vi "Type_3.vi"(7 "프런트패널 윈도우:동작":T1(ring)=enum."Default", 8 "에러 입력":errorcluster caption="에러 입력(에러 없음)", 11 "세부분류코드":string caption="확장자없는 파일 이름") -> (0 "error out":errorcluster)   [LabVIEW 2020]
uses:
  Support/Controls/Cmd_Mouse Popup.ctl
  Support/Controls/Clst_Query Info.ctl
  Support/Controls/Cmd_Read Query.ctl
  Support/Public/Polymorph/Array Dedup_1D Str.vi
  Support/Public/Polymorph/Cell Space_Table.vi
  <vilib>/addons/database/NI_Database_API.lvlib
panel:
  in  "탭 컨트롤":enum32{"검색", "등록", "CMC"}(tab)
  in  "일부추가":bool
  in  "최소범위검색":bool
  in  "최소 범위 검색":dbl
  in  "Condition_2":i32(listbox) caption="최소 측정 범위"
  out "인정범위":string[][](table)
  out "SQL Quary 컬럼명":string
  out "Calfunc":string[][](array[string])
  out "모델정보":string[][](array[string])
  in  "옵션검색":bool
  in  "옵션 검색 조건":string(combo)
  in  "모델검색":bool
  in  "모델 검색 조건":string
  in  "최대범위검색":bool
  in  "최대 범위 검색":dbl
  in  "전체추가":bool
  out "소분류코드":string
  out "측정기명":string
  in  "Condition_1":i32(listbox) caption="최대 측정 범위"
  in  "모델 및 옵션 List":i32(listbox)
  out "Load Proc":string[][](table) caption="등록된 교정 Procedure"
  in  "교정기능":string(combo)
  in  "구분 2":string(combo) caption="엑셀파일명"
  in  "참고 버튼":bool
  in  "교정값":string
  in  "명목값":string caption="명목값 (호칭)"
  in  "추가단위":string(combo)="mg" caption="단위"
  in  "구분":string(combo) caption="측정방식"
  out "Func_ext ?":bool
  out "배열":u32[](array[numeric])
  in  "단위":string(combo)
  in  "변경 버튼":bool
  in  "등록 버튼":bool
  in  "교정점 추가 버튼":bool
  in  "교정점":string
  in  "Proc":string[][](table) caption="등록할 교정 Procedure"
  in  "형식":string
  in  "옵션":string
  in  "최소눈금":string(combo)
  in  "교정기능 2":string(combo) caption="교정기능"
  in  "표시방식":string(combo)
  out "CMC":string[][](table)
  # "항목정보"
  # "검색옵션"
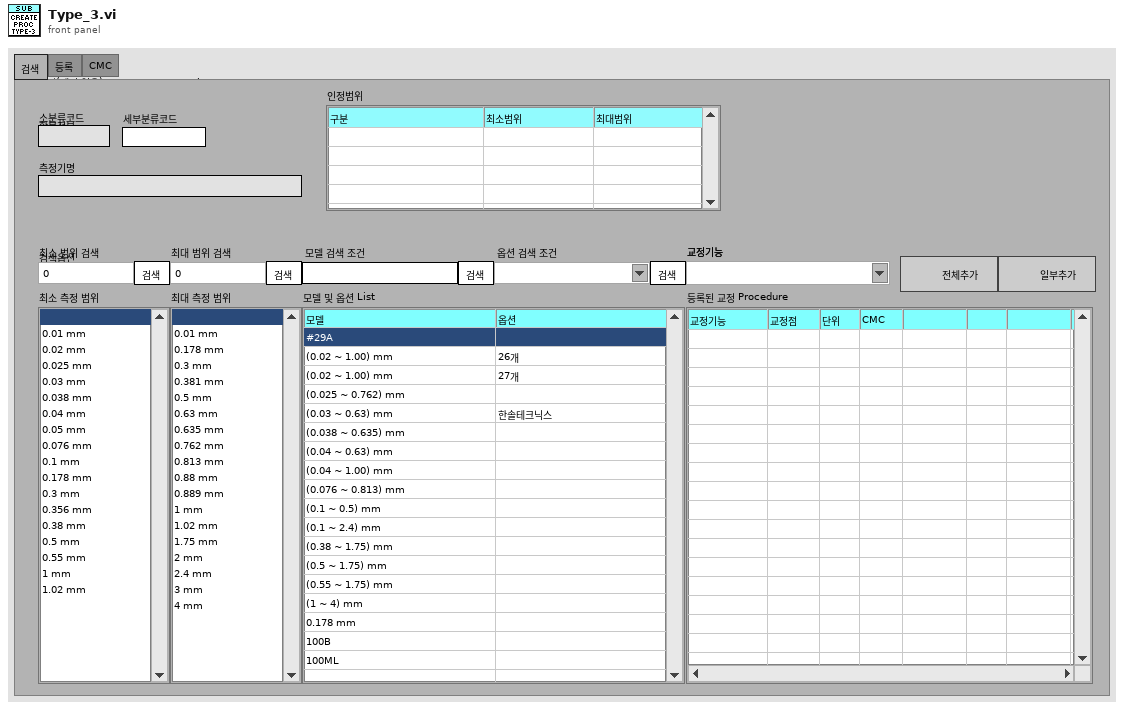
[diagram p1: front panel]
types:
  T1 = enum32{"Invalid", "Default", "Floating", "Floating/Auto-Hide", "Modal"}
  T2 = typedef "Cmd_Mouse Popup.ctl" = enum16{"활성화", "메뉴선택"}
  T3 = cluster{"Shift":bool, "Ctrl":bool, "Alt":bool, "Cmd":bool, "Opt":bool}
  T4 = typedef "Clst_Query Info.ctl" = cluster{"사번":string, "등록번호":string, "업체명":string, "세부분류코드":string, "형식":string, "기기번호":string, "FUNC":string, "FUNC_EXT":string, "옵션":string, "추가문자열":string, "일자":string, "배열 1":string[], "배열 2":string[], "항목명":string, "문자열":string, "이름":string}
  T5 = typedef "Cmd_Read Query.ctl" = enum16{"교정자 이름 얻기", "인증교정자 얻기", "기술책임자 얻기", "기책부책 얻기", "등록번호 얻기", "등록정보 얻기", "업체정보 얻기", "교정일자(CAMAS) 얻기", "교정일자(CALSTD) 얻기", "교정환경 얻기", "교정절차서 목록 얻기", "교정절차서명 얻기", "교정절차 목록얻기", "교정절차 얻기", "PROC 교정절차 얻기", "PROC SPEC 얻기", "교정절차(Func별) 얻기", "교정절차(Func_ext별) 얻기", "기관코드 얻기", "교정기능(세부분류) 얻기", "교정기능(모델) 얻기", "교정기능 목록 얻기", "교정기능 명칭 얻기", "교정기능 항목명칭 얻기", "DB (사용기준기) 얻기", "DB (기준기이름) 얻기", "DB (기준기이름목록) 얻기", "DB (기준기목록) 얻기", "DB (기준기값) 얻기", "DB (CMC) 얻기", "DB (FUNC) 얻기", "DB (CALNAME) 얻기", "DB (STDNAME) 얻기", "DB (SPEC) 얻기", "모델(항목전체) 얻기", "모델(최대범위) 얻기", "모델(최소범위) 얻기", "모델(최대최소) 얻기", "모델(범위조건) 얻기", "모델(등록요청) 얻기", "모델(형식별) 얻기", "모델(조건별) 얻기", "모델(모델검색) 얻기", "세부분류 목록 얻기", "기준기등록리스트 얻기", "STD Cal Date Check", "DB등록일자 얻기", "적용항목 얻기", "기타정보 얻기", "기준기요청 얻기", "서버버전 얻기"}
  T6 = cluster{refnum<vi>[], refnum<vi>[], refnum<vi>[], refnum<vi>[]}
  T7 = typedef "NI_Database_API.lvlib/Conn ObjectReference.ctl" = refnum<k1>
  T8 = typedef "LVRowAndColumnTypeDef.ctl" = cluster{"Row":i32, "Column":i32}
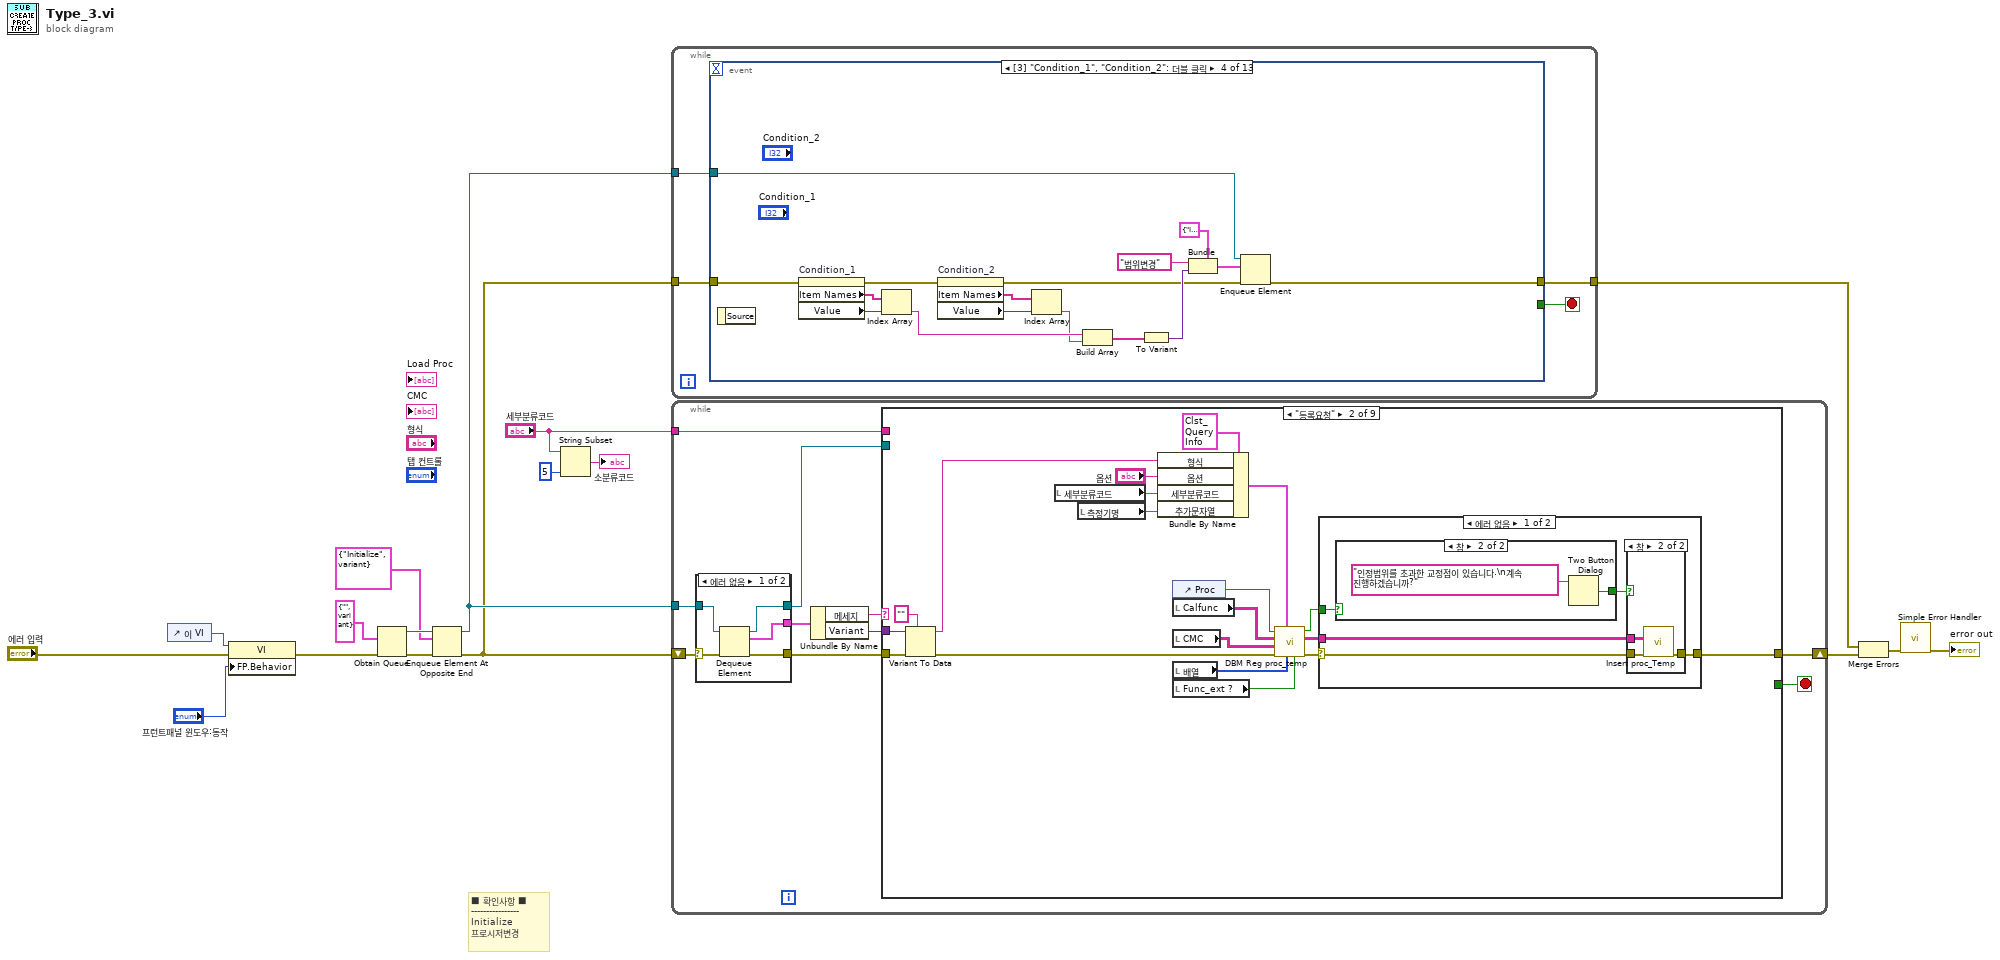
[diagram p0: block diagram]
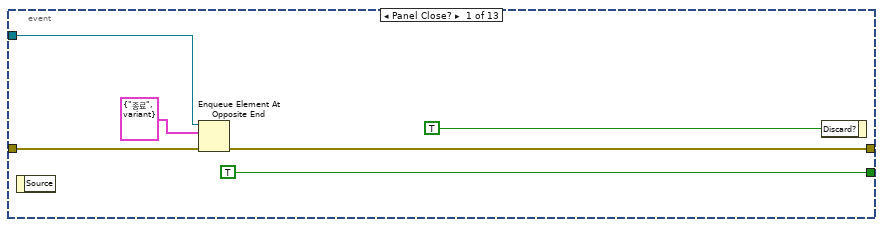
[diagram p2: hidden frame]
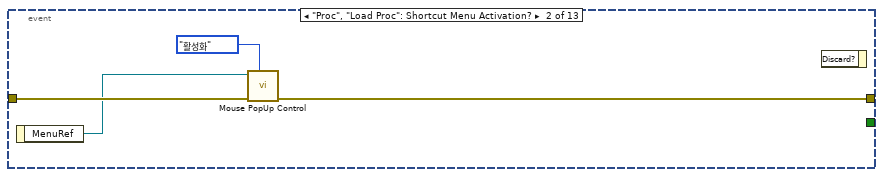
[diagram p3: hidden frame]
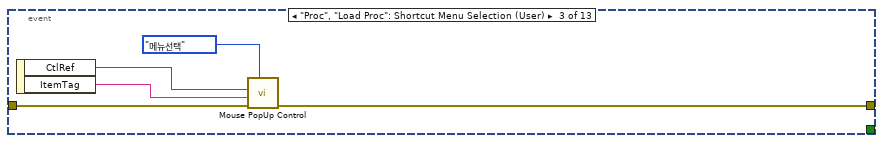
[diagram p4: hidden frame]
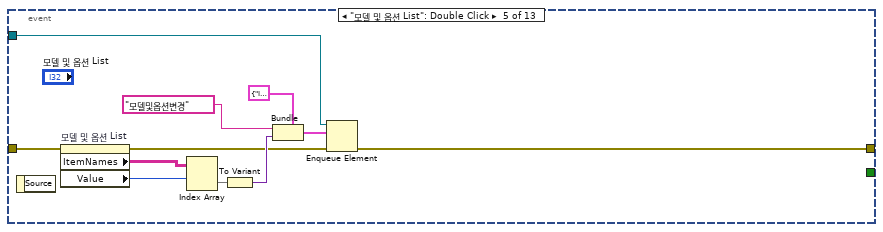
[diagram p5: hidden frame]
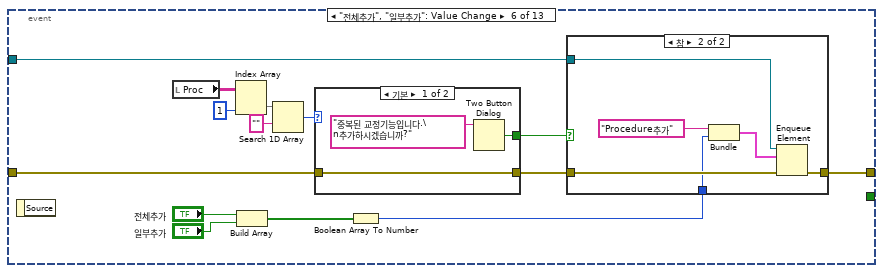
[diagram p6: hidden frame]
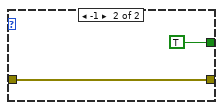
[diagram p8: hidden frame]
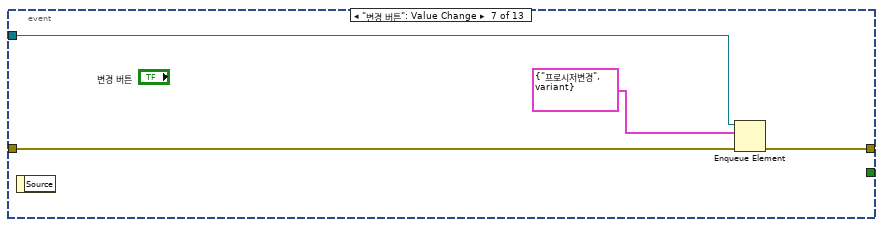
[diagram p9: hidden frame]
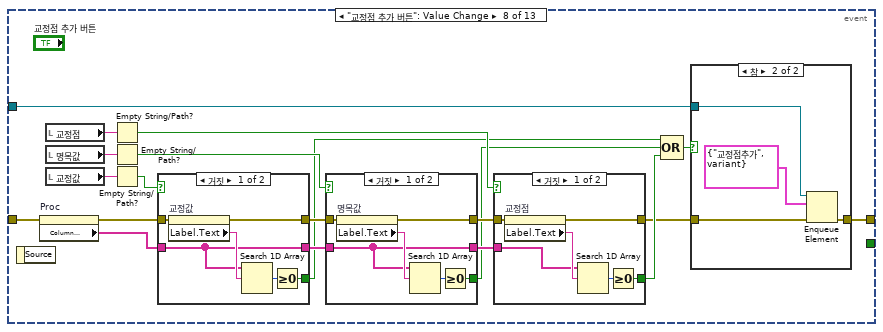
[diagram p10: hidden frame]
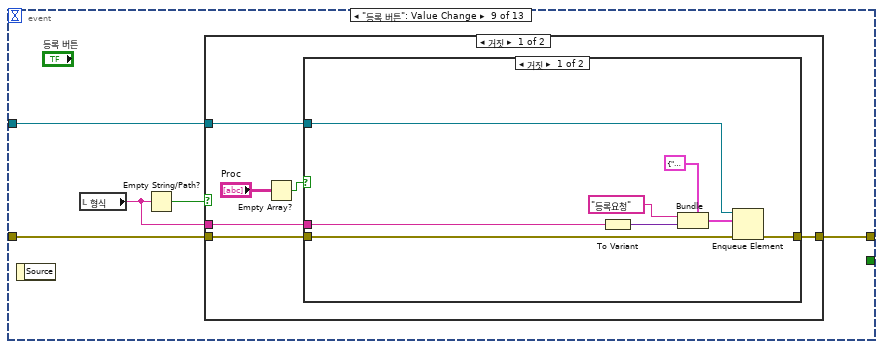
[diagram p15: hidden frame]
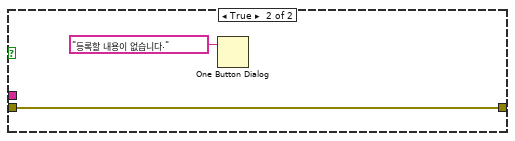
[diagram p16: hidden frame]
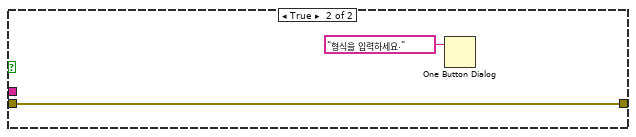
[diagram p17: hidden frame]
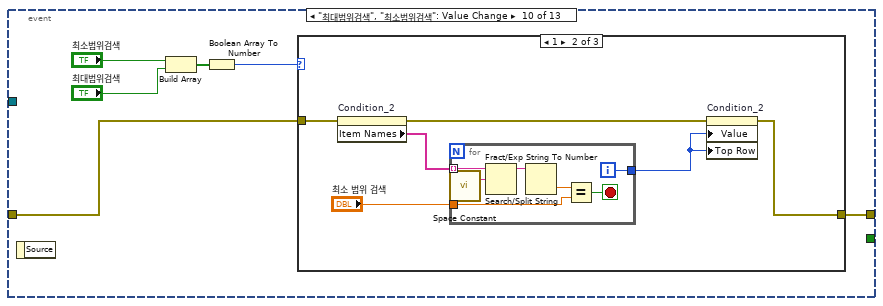
[diagram p18: hidden frame]
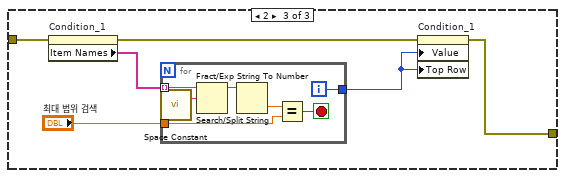
[diagram p20: hidden frame]
diagram:
  # "■ 확인사항 ■\n----------------\nInitialize\n프로시저변경"
  n1 = control-ref of="이 VI"() -> (w1:refnum<vi>)
  n2 = property class="VI"(reference=w1, error in="에러 입력", "FP.Behavior"="프런트패널 윈도우:동작") -> (error out=w7:errorcluster)  [unwired: 1 out]
  n3 = Obtain Queue(element data type=cluster{"메세지":string, "값":variant} {"메세지"="", "값"=variant} ("Message Cluster"), error in (no error)=w7) -> (queue out=w12:refnum<queue>, error out=w13:errorcluster)  [unwired: 3 in, 1 out]
  n4 = Enqueue Element At Opposite End(queue=w12, element=cluster{"메세지":string, "값":variant} {"메세지"="Initialize", "값"=variant} ("Message Cluster"), error in (no error)=w13) -> (queue out=w10:refnum<queue>, error out=w9:errorcluster)  [unwired: 1 in, 1 out]
  n5 = String Subset(string="세부분류코드", length (rest)=5 ("길이(나머지)")) -> (substring=→"소분류코드":string)  [unwired: 1 in]
  n6 = while {
    tunnel: w10 -> [w21]
    tunnel: w9 -> [w20]
    tunnel: [w19] -> w16
    stop <- w18 stop-if-true
    n7 = event shown="[3] \"Condition_1\", \"Condition_2\": 더블 클릭" {
      selector: _ -> [_ _ _ _ _ _ _ _ _ _ _ _ _]
      dyn-events: _ -> [_ _ _ _ _ _ _ _ _ _ _ _ _]
      timeout: _ -> [_ _ _ _ _ _ _ _ _ _ _ _ _]
      tunnel: w21 -> [w23 _ _ w51 w62 w76 w92 w112 w144 _ _ _ _]
      tunnel: w20 -> [w25 w31 w36 w50 w56 w75 w91 w111 w146 w170 w199 w223 _]
      tunnel: [w24 w30 w35 w52 w63 w77 w93 w113 w145 w169 w204 w222 _] -> w19
      tunnel: [TRUE ("우선순위 메시지?") _ _ _ _ _ _ _ _ _ _ _ _] -> w18
      event Panel Close? {
        n8 = event-data() -> ()  [unwired: 1 in, 1 out]
        n9 = Enqueue Element At Opposite End(queue=w23, element=cluster{"메세지":string, "값":variant} {"메세지"="종료", "값"=variant} ("원소"), error in (no error)=w25) -> (error out=w24:errorcluster)  [unwired: 1 in, 2 out]
        n10 = event-data("Discard?"=TRUE ("버림?")) -> ()  [unwired: 1 in, 1 out]
      }
      event "Proc", "Load Proc": Shortcut Menu Activation? {
        n11 = event-data() -> ("MenuRef"=w28:refnum<k9>)  [unwired: 1 in]
        n12 = call "Mouse PopUp Control.vi"("type"=Cmd_Mouse_Popup."활성화", "error in"=w31, "메뉴 참조"=w28) -> ("error out"=w30:errorcluster)  [unwired: 8 in]
        n13 = event-data() -> ()  [unwired: 2 in, 1 out]
      }
      event "Proc", "Load Proc": Shortcut Menu Selection (User) {
        n14 = event-data() -> ("CtlRef"=w32:refnum<vi>, "ItemTag"=w33:string)  [unwired: 1 in]
        n15 = call "Mouse PopUp Control.vi"("type"=Cmd_Mouse_Popup."메뉴선택", "error in"=w36, "아이템 태그"=w33, "Tbl 참조 번호"=w32) -> ("error out"=w35:errorcluster)  [unwired: 7 in]
      }
      event "Condition_1", "Condition_2": Double Click {
        n16 = event-data() -> ()  [unwired: 1 in, 1 out]
        n17 = property on="Condition_1" class="LstBox (엄격한)"(error in=w50) -> (error out=w43:errorcluster, "Item Names"=w47:string[], "Value"=w46:i32)  [unwired: 1 in, 1 out]
        n18 = Index Array(array=w47, index=w46) -> (element=w39:string)
        n19 = property on="Condition_2" class="LstBox (엄격한)"(error in=w43) -> (error out=w41:errorcluster, "Item Names"=w42:string[], "Value"=w40:i32)  [unwired: 1 in, 1 out]
        n20 = Index Array(array=w42, index=w40) -> (element=w38:string)
        n21 = Build Array(w39, w38) -> (w37:string[])
        n22 = To Variant(anything=w37) -> (Variant=w45:variant)
        n23 = Bundle(cluster=cluster{"메세지":string, "값":variant} {"메세지"="Initialize", "값"=variant} ("Message Cluster"), "메세지"="범위변경", "값"=w45) -> (w44:cluster{"메세지":string, "값":variant})
        n24 = Enqueue Element(queue=w51, element=w44, error in (no error)=w41) -> (error out=w52:errorcluster)  [unwired: 1 in, 2 out]
      }
      event "모델 및 옵션 List": Double Click {
        n25 = event-data() -> ()  [unwired: 1 in, 1 out]
        n26 = property on="모델 및 옵션 List" class="MCListbox (엄격한)"(error in=w56) -> (error out=w55:errorcluster, "ItemNames"=w54:string[][], "Value"=w53:i32)  [unwired: 1 in, 1 out]
        n27 = Index Array(array=w54, index (row)=w53) -> (element=w59:string[])  [unwired: 1 in]
        n28 = To Variant(anything=w59) -> (Variant=w58:variant)
        n29 = Bundle(cluster=cluster{"메세지":string, "값":variant} {"메세지"="Initialize", "값"=variant} ("Message Cluster"), "메세지"="모델및옵션변경", "값"=w58) -> (w57:cluster{"메세지":string, "값":variant})
        n30 = Enqueue Element(queue=w62, element=w57, error in (no error)=w55) -> (error out=w63:errorcluster)  [unwired: 1 in, 2 out]
      }
      event "전체추가", "일부추가": Value Change {
        n31 = event-data() -> ()  [unwired: 1 in, 1 out]
        n32 = local read "Proc"() -> (w72:string[][])
        n33 = Index Array(array=w72, index (col)=1 ("비활성화된 인덱스 (열)")) -> (element=w74:string[])  [unwired: 1 in]
        n34 = Build Array("전체추가", "일부추가") -> (w67:bool[])
        n35 = Search 1D Array(1D array=w74, element="" ("원소")) -> (index of element=w71:i32)  [unwired: 1 in]
        n36 = case shown="기본" w71 {
          tunnel: [w87 w88] -> w70
          tunnel: w75 -> [w87 w88]
          tunnel: [w85 TRUE ("T button?")] -> w69
          frame Default {
            n37 = Two Button Dialog(message="중복된 교정기능입니다.\n추가하시겠습니까?" ("메시지")) -> (T button?=w85:bool)  [unwired: 2 in]
          }
          frame -1 {
          }
        }
        n38 = Boolean Array To Number(Boolean array=w67) -> (number=w64:u32)
        n39 = case shown="참" w69 {
          tunnel: w76 -> [_ w84]
          tunnel: w70 -> [w78 w83]
          tunnel: [w78 w82] -> w77
          tunnel: w64 -> [_ w79]
          frame False {
          }
          frame True {
            n40 = Bundle("메세지"="Procedure추가", w79) -> (w81:cluster{"메세지":string, u32})  [unwired: 1 in]
            n41 = Enqueue Element(queue=w84, element=w81, error in (no error)=w83) -> (error out=w82:errorcluster)  [unwired: 1 in, 2 out]
          }
        }
      }
      event "변경 버튼": Value Change {
        n42 = event-data() -> ()  [unwired: 1 in, 1 out]
        n43 = Enqueue Element(queue=w92, element=cluster{"메세지":string, "값":variant} {"메세지"="프로시저변경", "값"=variant} ("Message Cluster"), error in (no error)=w91) -> (error out=w93:errorcluster)  [unwired: 1 in, 2 out]
      }
      event "교정점 추가 버튼": Value Change {
        n44 = event-data() -> ()  [unwired: 1 in, 1 out]
        n45 = property on="Proc" class="Tbl (엄격한)"(error in=w111) -> (error out=w101:errorcluster, "Column Headers[]"=w100:string[])  [unwired: 1 in, 1 out]
        n46 = local read "교정점"() -> (w110:string)
        n47 = local read "명목값"() -> (w107:string)
        n48 = local read "교정값"() -> (w106:string)
        n49 = Empty String/Path?(string/path=w110) -> (empty?=w105:bool)
        n50 = Empty String/Path?(string/path=w107) -> (empty?=w97:bool)
        n51 = Empty String/Path?(string/path=w106) -> (empty?=w96:bool)
        n52 = case shown="거짓" w96 {
          tunnel: [w119 w121] -> w104
          tunnel: w100 -> [w114 w120]
          tunnel: [w116 _] -> w95
          tunnel: w101 -> [w115 w121]
          tunnel: [w114 w120] -> w99
          frame False {
            n53 = property on="교정값" class="Str"(error in=w115) -> (error out=w119:errorcluster, "Label.Text"=w117:string)  [unwired: 1 in, 1 out]
            n54 = Search 1D Array(1D array=w114, element=w117) -> (index of element=w118:i32)  [unwired: 1 in]
            n55 = Greater Or Equal To 0?(x=w118) -> (x >= 0?=w116:bool)
          }
          frame True {
          }
        }
        n56 = case shown="거짓" w97 {
          tunnel: [w127 w129] -> w102
          tunnel: w99 -> [w122 w128]
          tunnel: [w124 _] -> w94
          tunnel: w104 -> [w123 w129]
          tunnel: [w122 w128] -> w98
          frame False {
            n57 = property on="명목값" class="Str"(error in=w123) -> (error out=w127:errorcluster, "Label.Text"=w125:string)  [unwired: 1 in, 1 out]
            n58 = Search 1D Array(1D array=w122, element=w125) -> (index of element=w126:i32)  [unwired: 1 in]
            n59 = Greater Or Equal To 0?(x=w126) -> (x >= 0?=w124:bool)
          }
          frame True {
          }
        }
        n60 = case shown="거짓" w105 {
          tunnel: [w135 w136] -> w103
          tunnel: w98 -> [w132 _]
          tunnel: [w131 _] -> w109
          tunnel: w102 -> [w130 w136]
          frame False {
            n61 = property on="교정점" class="Str"(error in=w130) -> (error out=w135:errorcluster, "Label.Text"=w133:string)  [unwired: 1 in, 1 out]
            n62 = Search 1D Array(1D array=w132, element=w133) -> (index of element=w134:i32)  [unwired: 1 in]
            n63 = Greater Or Equal To 0?(x=w134) -> (x >= 0?=w131:bool)
          }
          frame True {
          }
        }
        n64 = Compound Arithmetic op=OR(w95, w94, w109) -> (w108:bool)
        n65 = case shown="참" w108 {
          tunnel: [w137 w141] -> w113
          tunnel: w112 -> [_ w140]
          tunnel: w103 -> [w137 w138]
          frame False {
          }
          frame True {
            n66 = Enqueue Element(queue=w140, element=cluster{"메세지":string, "값":variant} {"메세지"="교정점추가", "값"=variant} ("Message Cluster"), error in (no error)=w138) -> (error out=w141:errorcluster)  [unwired: 1 in, 2 out]
          }
        }
      }
      event "등록 버튼": Value Change {
        n67 = event-data() -> ()  [unwired: 1 in, 1 out]
        n68 = local read "형식"() -> (w142:string)
        n69 = Empty String/Path?(string/path=w142) -> (empty?=w143:bool)
        n70 = case shown="거짓" w143 {
          tunnel: w146 -> [w152 w164]
          tunnel: [w151 w164] -> w145
          tunnel: w144 -> [w150 _]
          tunnel: w142 -> [w149 _]
          frame False {
            n71 = Empty Array?(array="Proc") -> (empty?=w148:bool)
            n72 = case shown="거짓" w148 {
              tunnel: w152 -> [w160 w162]
              tunnel: [w159 w162] -> w151
              tunnel: w150 -> [w158 _]
              tunnel: w149 -> [w157 _]
              frame False {
                n73 = To Variant(anything=w157) -> (Variant=w154:variant)
                n74 = Bundle(cluster=cluster{"메세지":string, "값":variant} {"메세지"="", "값"=variant} ("원소"), "메세지"="등록요청", "값"=w154) -> (w155:cluster{"메세지":string, "값":variant})
                n75 = Enqueue Element(queue=w158, element=w155, error in (no error)=w160) -> (error out=w159:errorcluster)  [unwired: 1 in, 2 out]
              }
              frame True {
                n76 = One Button Dialog(message="등록할 내용이 없습니다." ("메시지")) -> ()  [unwired: 1 in, 1 out]
              }
            }
          }
          frame True {
            n77 = One Button Dialog(message="형식을 입력하세요." ("메시지")) -> ()  [unwired: 1 in, 1 out]
          }
        }
      }
      event "최대범위검색", "최소범위검색": Value Change {
        n78 = event-data() -> ()  [unwired: 1 in, 1 out]
        n79 = Build Array("최소범위검색", "최대범위검색") -> (w167:bool[])
        n80 = Boolean Array To Number(Boolean array=w167) -> (number=w166:u32)
        n81 = case shown="1" w166 {
          tunnel: w170 -> [w171 w177 w190]
          tunnel: [w171 w174 w187] -> w169
          frame Default {
          }
          frame 1 {
            n82 = property on="Condition_2" class="LstBox (엄격한)"(error in=w177) -> (error out=w175:errorcluster, "Item Names"=w176:string[])  [unwired: 1 in, 1 out]
            n83 = for {
              tunnel: w176 -> [w183] mode=indexing
              tunnel: "최소 범위 검색" -> [w179]
              tunnel: [w184] -> w173
              i -> [w184]
              stop <- w178 stop-if-true
              n84 = call <vilib>:"Space Constant.vi"() -> ("String"=w182:string)
              n85 = Search/Split String(string=w183, search string/char (-)=w182) -> (substring before match=w181:string)  [unwired: 1 in, 2 out]
              n86 = Fract/Exp String To Number(string=w181) -> (number=w180:dbl)  [unwired: 3 in, 1 out]
              n87 = Equal?(x=w180, y=w179) -> (x = y?=w178:bool)
            }
            n88 = property on="Condition_2" class="LstBox (엄격한)"(error in=w175, "Value"=w173, "Top Row"=w173) -> (error out=w174:errorcluster)  [unwired: 1 in, 1 out]
          }
          frame 2 {
            n89 = property on="Condition_1" class="LstBox (엄격한)"(error in=w190) -> (error out=w188:errorcluster, "Item Names"=w189:string[])  [unwired: 1 in, 1 out]
            n90 = for {
              tunnel: w189 -> [w196] mode=indexing
              tunnel: "최대 범위 검색" -> [w192]
              tunnel: [w197] -> w186
              i -> [w197]
              stop <- w191 stop-if-true
              n91 = call <vilib>:"Space Constant.vi"() -> ("String"=w195:string)
              n92 = Search/Split String(string=w196, search string/char (-)=w195) -> (substring before match=w194:string)  [unwired: 1 in, 2 out]
              n93 = Fract/Exp String To Number(string=w194) -> (number=w193:dbl)  [unwired: 3 in, 1 out]
              n94 = Equal?(x=w193, y=w192) -> (x = y?=w191:bool)
            }
            n95 = property on="Condition_1" class="LstBox (엄격한)"(error in=w188, "Value"=w186, "Top Row"=w186) -> (error out=w187:errorcluster)  [unwired: 1 in, 1 out]
          }
        }
      }
      event "모델검색", "옵션검색": Value Change {
        n96 = event-data() -> ()  [unwired: 1 in, 1 out]
        n97 = Build Array("모델검색", "옵션검색") -> (w202:bool[])
        n98 = Boolean Array To Number(Boolean array=w202) -> (number=w200:u32)
        n99 = case shown="2" w200 {
          tunnel: [_ 0 ("비활성화된 인덱스 (열)") 1 ("비활성화된 인덱스 (열)")] -> w207
          tunnel: [_ "모델 검색 조건" "옵션 검색 조건"] -> w206
          frame Default {
          }
          frame 1 {
          }
          frame 2 {
          }
        }
        n100 = local read "모델정보"() -> (w198:string[][])
        n101 = Index Array(array=w198, index (col)=w207) -> (element=w208:string[])  [unwired: 1 in]
        n102 = for {
          tunnel: w208 -> [w217] mode=indexing
          tunnel: w206 -> [w216]
          tunnel: w198 -> [w214] mode=indexing
          tunnel: [w214] -> w205 mode=indexing if=w213
          n103 = Search and Replace String(input string=w217, search string=w216) -> (offset past replacement=w215:i32)  [unwired: 6 in, 3 out]
          n104 = Greater Or Equal To 0?(x=w215) -> (x >= 0?=w213:bool)
        }
        n105 = property on="모델 및 옵션 List" class="MCListbox (엄격한)"(error in=w199, "ItemNames"=w205) -> (error out=w204:errorcluster)  [unwired: 1 in, 1 out]
      }
      event "Proc": Key Down; "Proc": Key Repeat {
        n106 = event-data() -> ("PlatMods"=w218:T3, "ScanCode"=w221:i16, "Mods.Num Pad"=w220:bool, "CtlRef"=w219:refnum<vi>)  [unwired: 1 in]
        n107 = call "Cursor Control.vi"("플랫폼 조합키"=w218, "참조"=w219, "Num Pad"=w220, "ScanCode"=w221, "error in"=w223) -> ("error out"=w222:errorcluster)  [unwired: 5 in, 1 out]
      }
      event "참고 버튼": Value Change {
        n108 = event-data() -> ()  [unwired: 1 in, 1 out]
        n109 = call "DBM Reference.vi"() -> ()  [unwired: 12 in]
      }
    }
  }
  n110 = while {
    tunnel: w10 -> [w231]
    shift-right: [w233] -> w17
    shift-left: w9 -> [w227]
    tunnel: "세부분류코드" -> [w224]
    stop <- w232 stop-if-true
    n111 = case shown="에러 없음" w227 {
      selector: w227 -> [w234 w239]
      tunnel: w231 -> [w238 w243]
      tunnel: [w237 _] -> w225
      tunnel: [w235 w243] -> w230
      tunnel: [w236 w242] -> w226
      frame No Error {
        n112 = Dequeue Element(queue=w238, error in (no error)=w234) -> (queue out=w235:refnum<queue>, element=w236:cluster{"메세지":string, "값":variant}, error out=w237:errorcluster)  [unwired: 1 in, 1 out]
      }
      frame Error {
        n113 = To Variant(anything=w239) -> (Variant=w240:variant)
        n114 = Bundle("에러", "Variant"=w240) -> (w242:cluster{string, "Variant":variant})  [unwired: 1 in]
      }
    }
    n115 = Unbundle By Name(w226) -> ("메세지"=w228:string, "Variant"=w229:variant)
    n116 = case shown="\"등록요청\"" w228 {
      tunnel: w225 -> [w299 w321 w354 w397 w405 w445 w624 w769 w774]
      tunnel: [w245 w311 w350 w392 w410 w449 w622 w769 w771] -> w233
      tunnel: w230 -> [_ _ _ _ _ _ _ _ _]
      tunnel: w229 -> [_ w320 w353 w396 w406 _ _ _ w772]
      tunnel: [_ _ _ _ _ _ _ TRUE _] -> w232
      tunnel: w224 -> [w255 _ _ _ _ _ w612 _ _]
      frame "Initialize", Default {
        w267 = 0 ("인덱스")
        w266 = ""
        w289 = ""
        w302 = string[][] [] ("Proc")
        n117 = control-ref of="모델 및 옵션 List"() -> (w303:refnum<vi>)
        n118 = control-ref of="CMC"() -> (w278:refnum<vi>)
        n119 = local write "교정기능 2"(w289) -> ()
        n120 = local write "최소눈금"(w289) -> ()
        n121 = local write "표시방식"(w289) -> ()
        n122 = local write "단위"(w289) -> ()
        n123 = local write "교정점"(w289) -> ()
        n124 = local write "명목값"(w289) -> ()
        n125 = local write "교정값"(w289) -> ()
        n126 = local write "추가단위"(w289) -> ()
        n127 = control-ref of="표시방식"() -> (w297:refnum<vi>)
        n128 = control-ref of="단위"() -> (w298:refnum<vi>)
        n129 = control-ref of="추가단위"() -> (w288:refnum<vi>)
        n130 = control-ref of="추가단위"() -> (w287:refnum<vi>)
        n131 = control-ref of="교정점"() -> (w284:refnum<vi>)
        n132 = control-ref of="명목값"() -> (w285:refnum<vi>)
        n133 = control-ref of="교정값"() -> (w286:refnum<vi>)
        n134 = Build Array(w303) -> (w300:refnum<vi>[])
        n135 = Build Array(w297, w298, w288) -> (w259:refnum<vi>[])
        n136 = call "Start Create Procedure.vi"("에러 입력(에러 없음)"=w299, "Model List"=w300, "세부분류코드"=w255, "CMC"=w278) -> ("에러 출력"=w260:errorcluster, "Calfunc"=w250:string[][], "CMC"=→"인정범위":string[][], "모델정보 배열"=w247:string[][], "모델 및 옵션"=→"모델정보":string[][])  [unwired: 2 in, 1 out]
        "Calfunc" <- w250
        n137 = Build Array(w284, w285, w286, w287) -> (w257:refnum<vi>[])
        n138 = Index Array(array=w247, index (col) #1=1 ("비활성화된 인덱스 (열)"), index (col) #2=5 ("비활성화된 인덱스 (열)")) -> (element #1=w273:string[], element #2=w276:string[], element #3=w271:string[])  [unwired: 4 in]
        n139 = call-poly "Array Deduplication.vi"("정렬?"=TRUE, "배열 in"=w273) -> ("배열 out"=w272:string[])  [unwired: 8 in, 1 out]
        n140 = call-poly "Array Deduplication.vi"("정렬?"=TRUE, "배열 in"=w276) -> ("배열 out"=w275:string[])  [unwired: 8 in, 1 out]
        n141 = call-poly "Array Deduplication.vi"("정렬?"=TRUE, "배열 in"=w271) -> ("배열 out"=w270:string[])  [unwired: 8 in, 1 out]
        n142 = Index Array(array=w250, index (row) #1=0 ("인덱스 (열)"), index (col) #1=4 ("비활성화된 인덱스 (열)"), index (col) #2=3 ("비활성화된 인덱스 (열)")) -> (element #1=→"측정기명":string, element #2=w252:string[])  [unwired: 1 in]
        n143 = control-ref of="Proc"() -> (w296:refnum<vi>)
        n144 = control-ref of="Load Proc"() -> (w295:refnum<vi>)
        n145 = property on="옵션 검색 조건" class="CmbBox"(error in=w260, "Strings[]"=w272) -> (error out=w268:errorcluster)  [unwired: 1 in, 1 out]
        n146 = Insert Into Array(array=w275, index=w267, new element=w266) -> (w274:string[])
        n147 = Insert Into Array(array=w270, index=w267, new element=w266) -> (w269:string[])
        n148 = control-ref of="교정기능 2"() -> (w283:refnum<vi>)
        n149 = control-ref of="최소눈금"() -> (w293:refnum<vi>)
        n150 = control-ref of="표시방식"() -> (w292:refnum<vi>)
        n151 = control-ref of="단위"() -> (w291:refnum<vi>)
        n152 = control-ref of="구분"() -> (w290:refnum<vi>)
        n153 = control-ref of="구분 2"() -> (w282:refnum<vi>)
        n154 = Build Array(w296, w295) -> (w258:refnum<vi>[])
        n155 = property on="Condition_1" class="LstBox (엄격한)"(error in=w268, "Item Names"=w274) -> (error out=w251:errorcluster)  [unwired: 1 in, 1 out]
        n156 = Build Array(w283, w293, w292, w291, w290, w282) -> (w256:refnum<vi>[])
        n157 = property on="교정기능" class="CmbBox"(error in=w251, "Strings[]"=w252) -> (error out=w253:errorcluster)  [unwired: 1 in, 1 out]
        n158 = Bundle(w259, w258, w257, w256) -> (w254:T6)  [unwired: 1 in]
        n159 = call "DBM Unit Set.vi"("분류코드"=w255, "에러 입력(에러 없음)"=w253, "교정기능 문자열[]"=w252, "참조"=w254) -> ("에러 출력"=w246:errorcluster, "SQL query 컬럼명"=→"SQL Quary 컬럼명":string, "Condition2 캡션"=w244:string)  [unwired: 5 in]
        n160 = property on="Condition_2" class="LstBox (엄격한)"(error in=w246, "Caption.Text"=w244, "Item Names"=w269) -> (error out=w245:errorcluster)  [unwired: 1 in, 1 out]
        n161 = local write "탭 컨트롤"(enum32{"검색", "등록", "CMC"}."검색" ("탭 컨트롤")) -> ()
        n162 = local write "Proc"(w302) -> ()
        n163 = local write "Load Proc"(w302) -> ()
      }
      frame "등록요청" {
        n164 = Variant To Data(error in=w321, type="", Variant=w320) -> (data=w317:string)  [unwired: 1 out]
        n165 = local read "세부분류코드"() -> (w315:string)
        n166 = local read "측정기명"() -> (w314:string)
        n167 = Bundle By Name(cluster=T4 {"사번"="", "등록번호"="", "업체명"="", "세부분류코드"="", "형식"="", "기기번호"="", "FUNC"="", "FUNC_EXT"="", "옵션"="", "추가문자열"="", "일자"="", "배열 1"=[], "배열 2"=[], "항목명"="", "문자열"="", "이름"=""} ("Query info"), "형식"=w317, "옵션"="옵션", "세부분류코드"=w315, "추가문자열"=w314) -> (w304:T4)
        n168 = control-ref of="Proc"() -> (w305:refnum<vi>)
        n169 = local read "Calfunc"() -> (w310:string[][])
        n170 = local read "CMC"() -> (w313:string[][])
        n171 = local read "배열"() -> (w309:u32[])
        n172 = local read "Func_ext ?"() -> (w308:bool)
        n173 = call "DBM Reg proc_temp.vi"("Calfunc ?"=w308, "배열"=w309, "Query info"=w304, "에러 입력"=w321, "CMC"=w313, "calfunc"=w310, "Proc 참조 in"=w305) -> ("에러 출력"=w312:errorcluster, "배열출력"=w307:string[][], "에러?"=w306:bool)  [unwired: 2 in]
        n174 = case shown="에러 없음" w312 {
          selector: w312 -> [w322 w334]
          tunnel: w306 -> [w326 _]
          tunnel: [w325 w334] -> w311
          tunnel: w307 -> [w324 _]
          frame No Error {
            n175 = case shown="참" w326 {
              tunnel: [TRUE ("T button?") w328] -> w323
              frame False {
              }
              frame True {
                n176 = Two Button Dialog(message="인정범위를 초과한 교정점이 있습니다.\n계속 진행하겠습니까?" ("메시지")) -> (T button?=w328:bool)  [unwired: 2 in]
              }
            }
            n177 = case shown="참" w323 {
              tunnel: [w330 w333] -> w325
              tunnel: w322 -> [w330 w332]
              tunnel: w324 -> [_ w331]
              frame False {
              }
              frame True {
                n178 = call "Insert proc_Temp.vi"("에러 입력(에러 없음)"=w332, "Proc 입력"=w331) -> ("에러 출력"=w333:errorcluster)  [unwired: 9 in]
              }
            }
          }
          frame Error {
          }
        }
      }
      frame "범위변경" {
        n179 = Variant To Data(error in=w354, type=string[] [], Variant=w353) -> (data=w337:string[], error out=w352:errorcluster)
        n180 = Index Array(array=w337) -> (element #1=w340:string, element #2=w339:string)  [unwired: 2 in]
        n181 = case shown="\"\"" w340 {
          selector: w340 -> [w356 w365]
          tunnel: w339 -> [w360 w368]
          tunnel: [w359 w367] -> w338
          tunnel: w337 -> [w358 _]
          tunnel: [w357 _] -> w336
          tunnel: [w355 w366] -> w335
          frame Default {
            n182 = case shown="\"\"" w360 {
              tunnel: [Cmd_Read_Query."모델(최대범위) 얻기" ("Query Command") Cmd_Read_Query."모델(최대최소) 얻기" ("Query Command")] -> w359
              tunnel: w358 -> [_ w363]
              tunnel: [_ w363] -> w357
              tunnel: w356 -> [w361 _]
              tunnel: [w361 _] -> w355
              frame "" {
              }
              frame Default {
              }
            }
          }
          frame "" {
            n183 = case shown="기본" w368 {
              selector: w368 -> [_ w371]
              tunnel: [Cmd_Read_Query."모델(최대범위) 얻기" ("Query Command") Cmd_Read_Query."모델(최소범위) 얻기" ("Query Command")] -> w367
              tunnel: [w369 w371] -> w366
              tunnel: w365 -> [w369 _]
              frame "" {
              }
              frame Default {
              }
            }
          }
        }
        n184 = local read "세부분류코드"() -> (w342:string)
        n185 = call "DB Open.vi"("에러 입력"=w352) -> ("에러 출력"=w349:errorcluster, "참조 번호 출력"=w346:T7)  [unwired: 9 in]
        n186 = Bundle By Name(cluster=T4 {"사번"="", "등록번호"="", "업체명"="", "세부분류코드"="", "형식"="", "기기번호"="", "FUNC"="", "FUNC_EXT"="", "옵션"="", "추가문자열"="", "일자"="", "배열 1"=[], "배열 2"=[], "항목명"="", "문자열"="", "이름"=""} ("Query info"), "세부분류코드"=w342, "배열 1"=w336, "추가문자열"=w335) -> (w343:T4)
        n187 = call "DB Read Queries.vi"("Query info"=w343, "Query Command"=w338, "에러 입력(에러 없음)"=w349, "참조 번호 입력"=w346) -> ("에러 출력"=w348:errorcluster, "Data"=w347:string[][], "참조 번호 출력"=w345:T7)  [unwired: 3 in, 2 out]
        n188 = call <vilib>:"DB Tools Close Connection.vi"("error in (no error)"=w348, "connection reference"=w345) -> ("error out"=w351:errorcluster)  [unwired: 5 in]
        n189 = property on="모델 및 옵션 List" class="MCListbox (엄격한)"(error in=w351, "ItemNames"=w347) -> (error out=w350:errorcluster)  [unwired: 1 in, 1 out]
      }
      frame "모델및옵션변경" {
        n190 = local read "세부분류코드"() -> (w384:string)
        n191 = Variant To Data(error in=w397, type=string[] [], Variant=w396) -> (data=w393:string[], error out=w395:errorcluster)
        n192 = Index Array(array=w393) -> (element #1=w383:string, element #2=w382:string)  [unwired: 2 in]
        n193 = Bundle By Name(cluster=T4 {"사번"="", "등록번호"="", "업체명"="", "세부분류코드"="", "형식"="", "기기번호"="", "FUNC"="", "FUNC_EXT"="", "옵션"="", "추가문자열"="", "일자"="", "배열 1"=[], "배열 2"=[], "항목명"="", "문자열"="", "이름"=""} ("Query info"), "세부분류코드"=w384, "형식"=w383, "옵션"=w382) -> (w381:T4)
        n194 = call "DB Open.vi"("에러 입력"=w395) -> ("에러 출력"=w390:errorcluster, "참조 번호 출력"=w388:T7)  [unwired: 9 in]
        n195 = local read "SQL Quary 컬럼명"() -> (w373:string)
        n196 = call "DB Read Queries.vi"("Query info"=w381, "Query Command"=Cmd_Read_Query."교정절차 얻기", "에러 입력(에러 없음)"=w390, "참조 번호 입력"=w388) -> ("에러 출력"=w389:errorcluster, "Data"=w380:string[][], "참조 번호 출력"=w387:T7)  [unwired: 3 in, 2 out]
        n197 = call <vilib>:"DB Tools Close Connection.vi"("error in (no error)"=w389, "connection reference"=w387) -> ("error out"=w378:errorcluster)  [unwired: 5 in]
        n198 = local read "Calfunc"() -> (w374:string[][])
        n199 = call "Condition Filter.vi"("Cal func in"=w374, "컬럼명"=w373, "error in (no error)"=w378, "Cal Proc in"=w380) -> ("error out"=w377:errorcluster, "배열"=→"배열":u32[], "Func_ext ?"=→"Func_ext ?":bool, "Cal Proc out"=w379:string[][])  [unwired: 4 in]
        n200 = control-ref of="Load Proc"() -> (w391:refnum<vi>)
        n201 = call-poly "Cell Spacing.vi"("error in"=w377, "Data in"=w379, "테이블 참조 in"=w391) -> ("error out"=w392:errorcluster)  [unwired: 6 in, 2 out]
      }
      frame "Procedure추가" {
        n202 = Variant To Data(error in=w405, type=u32 0 ("숫자"), Variant=w406) -> (data=w398:u32, error out=w404:errorcluster)
        n203 = local read "Func_ext ?"() -> (w403:bool)
        n204 = Empty String/Path?(string/path="교정기능") -> (empty?=w401:bool)
        n205 = local read "Load Proc"() -> (w411:string[][])
        n206 = Not(x=w403) -> (.not. x?=w399:bool)
        n207 = local write "탭 컨트롤"(enum32{"검색", "등록", "CMC"}."등록" ("탭 컨트롤")) -> ()
        n208 = Or(x=w401, y=w399) -> (x .or. y?=w400:bool)
        n209 = case shown="거짓" w400 {
          tunnel: [w419 w435] -> w414
          tunnel: w411 -> [w418 w435]
          tunnel: "교정기능" -> [w416 _]
          tunnel: w398 -> [w417 _]
          frame False {
            n210 = case shown="1, 기본" w417 {
              tunnel: [w421 w430] -> w419
              tunnel: w418 -> [w422 w429]
              tunnel: w416 -> [w420 w428]
              frame 2 {
                n211 = for {
                  tunnel: w422 -> [w427] mode=indexing
                  tunnel: w420 -> [w424]
                  tunnel: [w427] -> w421 mode=indexing if=w423
                  n212 = Index Array(array=w427, index=1 ("인덱스")) -> (element=w425:string)
                  n213 = Equal?(x=w425, y=w424) -> (x = y?=w423:bool)
                }
              }
              frame 1, Default {
                n214 = for {
                  tunnel: w429 -> [w434] mode=indexing
                  tunnel: w428 -> [w431]
                  tunnel: [w433] -> w430 mode=indexing
                  n215 = Replace Array Subset(array=w434, new element=w431, index=1 ("인덱스")) -> (w433:string[])
                }
              }
            }
          }
          frame True {
          }
        }
        n216 = local read "Proc"() -> (w415:string[][])
        n217 = Empty Array?(array=w415) -> (empty?=w413:bool)
        n218 = case shown="거짓" w413 {
          tunnel: w415 -> [w438 _]
          tunnel: w414 -> [w437 w439]
          tunnel: [w436 w439] -> w408
          frame False {
            n219 = Insert Into Array(array=w438, new element=w437) -> (w436:string[][])  [unwired: 2 in]
          }
          frame True {
          }
        }
        n220 = control-ref of="Proc"() -> (w409:refnum<vi>)
        n221 = call-poly "Cell Spacing.vi"("error in"=w404, "Data in"=w408, "테이블 참조 in"=w409) -> ("error out"=w410:errorcluster)  [unwired: 6 in, 2 out]
      }
      frame "프로시저변경" {
        n222 = property on="Proc" class="Tbl (엄격한)"(error in=w445) -> (error out=w466:errorcluster, "Column Headers[]"=w448:string[], "Selection Size"=w444:T8, "Selection Start"=w443:T8)  [unwired: 1 in, 1 out]
        n223 = local read "Proc"() -> (w471:string[][])
        n224 = Unbundle By Name(w444) -> ("Row"=w441:i32)
        n225 = Unbundle By Name(w443) -> ("Row"=w440:i32)
        n226 = Add(x=w441, y=w440) -> (x+y=w442:i32)
        n227 = property on="최소눈금" class="CmbBox"(error in=w466) -> (error out=w463:errorcluster, "Label.Text"=w465:string)  [unwired: 1 in, 1 out]
        n228 = property on="단위" class="CmbBox"(error in=w463) -> (error out=w459:errorcluster, "Label.Text"=w462:string)  [unwired: 1 in, 1 out]
        n229 = Search 1D Array(1D array=w448, element=w465) -> (index of element=w464:i32)  [unwired: 1 in]
        n230 = Search 1D Array(1D array=w448, element=w462) -> (index of element=w461:i32)  [unwired: 1 in]
        n231 = Increment(x=w461) -> (x+1=w456:i32)
        n232 = property on="표시방식" class="CmbBox"(error in=w459) -> (error out=w454:errorcluster, "Label.Text"=w458:string)  [unwired: 1 in, 1 out]
        n233 = Search 1D Array(1D array=w448, element=w462, start index (0)=w456) -> (index of element=w460:i32)
        n234 = property on="구분" class="CmbBox"(error in=w454) -> (error out=w450:errorcluster, "Caption.Text"=w453:string)  [unwired: 1 in, 1 out]
        n235 = Search 1D Array(1D array=w448, element=w458) -> (index of element=w457:i32)  [unwired: 1 in]
        n236 = property on="구분 2" class="CmbBox"(error in=w450) -> (error out=w449:errorcluster, "Caption.Text"=w447:string)  [unwired: 1 in, 1 out]
        n237 = Search 1D Array(1D array=w448, element=w453) -> (index of element=w452:i32)  [unwired: 1 in]
        n238 = Search 1D Array(1D array=w448, element=w447) -> (index of element=w446:i32)  [unwired: 1 in]
        n239 = for {
          tunnel: w471 -> [w491] mode=indexing
          tunnel: "최소눈금" -> [w493]
          tunnel: [w492] -> w470 mode=indexing
          tunnel: "교정기능 2" -> [w489]
          tunnel: "단위" -> [w490]
          tunnel: "표시방식" -> [w488]
          tunnel: w464 -> [w487]
          tunnel: w461 -> [w486]
          tunnel: w460 -> [w485]
          tunnel: w457 -> [w484]
          tunnel: "구분" -> [w483]
          tunnel: w452 -> [w482]
          tunnel: "구분 2" -> [w481]
          tunnel: w446 -> [w480]
          tunnel: w441 -> [w476]
          tunnel: w440 -> [w474]
          tunnel: w442 -> [w473]
          i -> [w475]
          n240 = In Range and Coerce(upper limit=w473, x=w475, lower limit=w474) -> (In Range?=w478:bool)  [unwired: 1 out]
          n241 = Equal To 0?(x=w476) -> (x = 0?=w479:bool)
          n242 = Or(x=w479, y=w478) -> (x .or. y?=w477:bool)
          n243 = case shown="참" w477 {
            tunnel: w493 -> [_ w508]
            tunnel: [w494 w507] -> w492
            tunnel: w491 -> [w494 w506]
            tunnel: w490 -> [_ w505]
            tunnel: w489 -> [_ w504]
            tunnel: w488 -> [_ w503]
            tunnel: w487 -> [_ w502]
            tunnel: w486 -> [_ w501]
            tunnel: w485 -> [_ w500]
            tunnel: w484 -> [_ w499]
            tunnel: w483 -> [_ w498]
            tunnel: w482 -> [_ w497]
            tunnel: w481 -> [_ w496]
            tunnel: w480 -> [_ w495]
            frame False {
            }
            frame True {
              n244 = case shown="기본" w504 {
                selector: w504 -> [w522 _]
                tunnel: w508 -> [w520 w583]
                tunnel: [w524 w585] -> w507
                tunnel: w506 -> [w521 w584]
                tunnel: w505 -> [w519 w582]
                tunnel: w503 -> [w517 w581]
                tunnel: w502 -> [w516 w580]
                tunnel: w501 -> [w515 w579]
                tunnel: w500 -> [w514 w578]
                tunnel: w499 -> [w513 w577]
                tunnel: w498 -> [w512 w576]
                tunnel: w497 -> [w511 w575]
                tunnel: w496 -> [w509 w573]
                tunnel: w495 -> [w510 w574]
                frame Default {
                  n245 = Index Array(array=w521) -> (element #2=w523:string)  [unwired: 2 in, 1 out]
                  n246 = Equal?(x=w523, y=w522) -> (x = y?=w518:bool)
                  n247 = case shown="참" w518 {
                    tunnel: [w525 w527] -> w524
                    tunnel: w521 -> [w525 w542]
                    tunnel: w520 -> [_ w540]
                    tunnel: w519 -> [_ w539]
                    tunnel: w517 -> [_ w537]
                    tunnel: w516 -> [_ w536]
                    tunnel: w515 -> [_ w535]
                    tunnel: w514 -> [_ w534]
                    tunnel: w513 -> [_ w533]
                    tunnel: w512 -> [_ w531]
                    tunnel: w511 -> [_ w530]
                    tunnel: w510 -> [_ w529]
                    tunnel: w509 -> [_ w526]
                    frame False {
                    }
                    frame True {
                      n248 = case shown="기본" w540 {
                        selector: w540 -> [_ w560]
                        tunnel: [w558 w562] -> w541
                        tunnel: w542 -> [w558 w561]
                        tunnel: w536 -> [_ w559]
                        frame "" {
                        }
                        frame Default {
                          n249 = Replace Array Subset(array=w561, new element=w560, index=w559) -> (w562:string[])
                        }
                      }
                      n250 = case shown="기본" w539 {
                        selector: w539 -> [_ w566]
                        tunnel: [w563 w568] -> w538
                        tunnel: w541 -> [w563 w567]
                        tunnel: w535 -> [_ w565]
                        tunnel: w534 -> [_ w564]
                        frame "" {
                        }
                        frame Default {
                          n251 = Replace Array Subset(array=w567, new element #1=w566, index #1=w565, new element #2=w566, index #2=w564) -> (w568:string[])
                        }
                      }
                      n252 = case shown="기본" w537 {
                        selector: w537 -> [_ w555]
                        tunnel: [w553 w557] -> w532
                        tunnel: w538 -> [w553 w556]
                        tunnel: w533 -> [_ w554]
                        frame "" {
                        }
                        frame Default {
                          n253 = Replace Array Subset(array=w556, new element=w555, index=w554) -> (w557:string[])
                        }
                      }
                      n254 = case shown="기본" w531 {
                        selector: w531 -> [_ w550]
                        tunnel: [w548 w552] -> w528
                        tunnel: w532 -> [w548 w551]
                        tunnel: w530 -> [_ w549]
                        frame "" {
                        }
                        frame Default {
                          n255 = Replace Array Subset(array=w551, new element=w550, index=w549) -> (w552:string[])
                        }
                      }
                      n256 = case shown="기본" w526 {
                        selector: w526 -> [_ w545]
                        tunnel: [w543 w547] -> w527
                        tunnel: w528 -> [w543 w546]
                        tunnel: w529 -> [_ w544]
                        frame "" {
                        }
                        frame Default {
                          n257 = Replace Array Subset(array=w546, new element=w545, index=w544) -> (w547:string[])
                        }
                      }
                    }
                  }
                }
                frame "" {
                  n258 = case shown="기본" w583 {
                    selector: w583 -> [_ w603]
                    tunnel: [w601 w605] -> w572
                    tunnel: w584 -> [w601 w604]
                    tunnel: w580 -> [_ w602]
                    frame "" {
                    }
                    frame Default {
                      n259 = Replace Array Subset(array=w604, new element=w603, index=w602) -> (w605:string[])
                    }
                  }
                  n260 = case shown="기본" w582 {
                    selector: w582 -> [_ w609]
                    tunnel: [w606 w611] -> w571
                    tunnel: w572 -> [w606 w610]
                    tunnel: w579 -> [_ w608]
                    tunnel: w578 -> [_ w607]
                    frame "" {
                    }
                    frame Default {
                      n261 = Replace Array Subset(array=w610, new element #1=w609, index #1=w608, new element #2=w609, index #2=w607) -> (w611:string[])
                    }
                  }
                  n262 = case shown="기본" w581 {
                    selector: w581 -> [_ w598]
                    tunnel: [w596 w600] -> w570
                    tunnel: w571 -> [w596 w599]
                    tunnel: w577 -> [_ w597]
                    frame "" {
                    }
                    frame Default {
                      n263 = Replace Array Subset(array=w599, new element=w598, index=w597) -> (w600:string[])
                    }
                  }
                  n264 = case shown="기본" w576 {
                    selector: w576 -> [_ w593]
                    tunnel: [w591 w595] -> w569
                    tunnel: w570 -> [w591 w594]
                    tunnel: w575 -> [_ w592]
                    frame "" {
                    }
                    frame Default {
                      n265 = Replace Array Subset(array=w594, new element=w593, index=w592) -> (w595:string[])
                    }
                  }
                  n266 = case shown="기본" w573 {
                    selector: w573 -> [_ w588]
                    tunnel: [w586 w590] -> w585
                    tunnel: w569 -> [w586 w589]
                    tunnel: w574 -> [_ w587]
                    frame "" {
                    }
                    frame Default {
                      n267 = Replace Array Subset(array=w589, new element=w588, index=w587) -> (w590:string[])
                    }
                  }
                }
              }
            }
          }
        }
        n268 = local write "Proc"(w470) -> ()
      }
      frame "교정점추가" {
        w616 = "단위" ("원소")
        n269 = property on="Proc" class="Tbl (엄격한)"(error in=w624) -> (error out=w623:errorcluster, "Column Headers[]"=w617:string[], "Value"=w630:string[][], "Selection Start"=w631:T8)  [unwired: 1 in, 1 out]
        n270 = Unbundle(w631) -> ("Row"=w629:i32)  [unwired: 1 out]
        n271 = property on="교정점" class="Str"(error in=w623) -> (error out=w618:errorcluster, "Label.Text"=w628:string)  [unwired: 1 in, 1 out]
        n272 = Search 1D Array(1D array=w617, element=w628) -> (index of element=w621:i32)  [unwired: 1 in]
        n273 = Search 1D Array(1D array=w617, element=w616) -> (index of element=w615:i32)  [unwired: 1 in]
        n274 = Increment(x=w615) -> (x+1=w614:i32)
        n275 = Search 1D Array(1D array=w617, element=w616, start index (0)=w614) -> (index of element=w613:i32)
        n276 = property on="명목값" class="Str"(error in=w618) -> (error out=w626:errorcluster, "Label.Text"=w627:string)  [unwired: 1 in, 1 out]
        n277 = Search 1D Array(1D array=w617, element=w627) -> (index of element=w620:i32)  [unwired: 1 in]
        n278 = property on="교정값" class="Str"(error in=w626) -> (error out=w622:errorcluster, "Label.Text"=w625:string)  [unwired: 1 in, 1 out]
        n279 = Search 1D Array(1D array=w617, element=w625) -> (index of element=w619:i32)  [unwired: 1 in]
        n280 = case shown="기본" w629 {
          selector: w629 -> [_ w644]
          tunnel: w630 -> [_ w649]
          tunnel: w621 -> [_ w643]
          tunnel: w615 -> [_ w637]
          tunnel: w620 -> [_ w635]
          tunnel: w619 -> [_ w636]
          tunnel: w613 -> [_ w638]
          tunnel: w612 -> [_ w634]
          frame 0 {
          }
          frame Default {
            n281 = Decrement(x=w644) -> (x-1=w645:i32)
            n282 = Index Array(array=w649, index (col) #1=4 ("비활성화된 인덱스 (열)"), index (row) #2=w645) -> (element #1=w632:string[], element #2=w648:string[])  [unwired: 2 in]
            n283 = case shown="기본" w634 {
              tunnel: w648 -> [w670 w690 w717]
              tunnel: "교정점" -> [_ w688 w716]
              tunnel: w643 -> [_ w687 w715]
              tunnel: [w671 w691 w713] -> w642
              tunnel: "추가단위" -> [w650 w689 w709]
              tunnel: "명목값" -> [w652 _ w708]
              tunnel: "교정값" -> [w651 _ w707]
              tunnel: w638 -> [_ _ w706]
              tunnel: w637 -> [_ _ w705]
              tunnel: w636 -> [_ _ w704]
              tunnel: w635 -> [_ _ w703]
              tunnel: w632 -> [_ _ _]
              frame "20116-2" {
                w659 = dbl[] [1.0, 2.0, 5.0, 10.0, 20.0, 50.0, 100.0, 200.0, 500.0, 1000.0, 2000.0, 5000.0, 10000.0, 20000.0, 50000.0]
                n284 = case shown="\"N\"" w650 {
                  tunnel: [1.0 1e-06 0.001 1.0 1000.0 1000000.0 28.34952 453.5924 101.9716] -> w653
                  frame Default {
                  }
                  frame "μg" {
                  }
                  frame "mg" {
                  }
                  frame "g" {
                  }
                  frame "kg" {
                  }
                  frame "ton" {
                  }
                  frame "oz" {
                  }
                  frame "lb" {
                  }
                  frame "N" {
                  }
                }
                n285 = Fract/Exp String To Number(string=w651) -> (number=w655:dbl)  [unwired: 3 in, 1 out]
                n286 = Multiply(x=w655, y=w653) -> (x*y=w654:dbl)
                n287 = for {
                  tunnel: w654 -> [w686]
                  tunnel: w659 -> [w685] mode=indexing
                  tunnel: [w683] -> w660
                  i -> [w683]
                  stop <- w684 stop-if-true
                  n288 = Less?(x=w686, y=w685) -> (x < y?=w684:bool)
                }
                n289 = Decrement(x=w660) -> (x-1=w661:i32)
                n290 = Index Array(array=w659, index #1=w661) -> (element #1=w666:dbl, element #2=w667:dbl)  [unwired: 1 in]
                n291 = Add(x=w666, y=w667) -> (x+y=w662:dbl)
                n292 = Divide(x=w662, y=2.0) -> (x/y=w664:dbl)
                n293 = Greater Or Equal?(x=w664, y=w654) -> (x >= y?=w665:bool)
                n294 = Format Into String(format string="%#.6f" ("포맷 문자열"), w654) -> (resulting string=w656:string)  [unwired: 2 in, 1 out]
                n295 = Select(t=w666, s=w665, f=w667) -> (s? t:f=w669:dbl)
                n296 = Format Into String(format string="%.0f" ("포맷 문자열"), w669) -> (resulting string=w658:string)  [unwired: 2 in, 1 out]
                n297 = Replace Array Subset(array=w670, new element #1=w652, index #1=2 ("인덱스"), new element #2=w651, new element #3=w650, new element #4=w656, new element #5=w658, new element #6="g") -> (w671:string[])  [unwired: 5 in]
              }
              frame "20414-0" {
                n298 = Multiply(x=9.80665, y=0.9991026) -> (x*y=w698:dbl)
                n299 = call "Unit Conversion.vi"("환산단위"="kPa", "입력단위"=w689, "입력값"=w688) -> ("환산단위"=w693:string, "환산값 (DBL)"=w697:dbl, "환산값 (string)"=w692:string)  [unwired: 3 in, 3 out]
                n300 = Divide(x=w697, y=w698) -> (x/y=w699:dbl)
                n301 = Format Into String(format string="%.2f" ("포맷 문자열"), w699) -> (resulting string=w701:string)  [unwired: 2 in, 1 out]
                n302 = Replace Array Subset(array=w690, new element #1=w692, index #1=w687, new element #2=w693, new element #3=w701, index #3=2 ("인덱스")) -> (w691:string[])  [unwired: 1 in]
              }
              frame Default {
                n303 = case shown="기본" w715 {
                  selector: w715 -> [_ w760]
                  tunnel: w717 -> [w758 w762]
                  tunnel: w716 -> [_ w759]
                  tunnel: [w758 w761] -> w712
                  frame -1 {
                  }
                  frame Default {
                    n304 = case shown="기본" w759 {
                      selector: w759 -> [_ w764]
                      tunnel: w762 -> [w763 w767]
                      tunnel: [w763 w766] -> w761
                      tunnel: w760 -> [_ w765]
                      frame "" {
                      }
                      frame Default {
                        n305 = Replace Array Subset(array=w767, new element=w764, index=w765) -> (w766:string[])
                      }
                    }
                  }
                }
                n306 = case shown="기본" w705 {
                  selector: w705 -> [_ w750]
                  tunnel: w712 -> [w748 w752]
                  tunnel: w709 -> [_ w749]
                  tunnel: [w748 w751] -> w711
                  frame -1 {
                  }
                  frame Default {
                    n307 = case shown="기본" w749 {
                      selector: w749 -> [_ w754]
                      tunnel: w752 -> [w753 w757]
                      tunnel: [w753 w756] -> w751
                      tunnel: w750 -> [_ w755]
                      frame "" {
                      }
                      frame Default {
                        n308 = Replace Array Subset(array=w757, new element=w754, index=w755) -> (w756:string[])
                      }
                    }
                  }
                }
                n309 = case shown="기본" w706 {
                  selector: w706 -> [_ w740]
                  tunnel: w711 -> [w738 w742]
                  tunnel: w709 -> [_ w739]
                  tunnel: [w738 w741] -> w710
                  frame -1 {
                  }
                  frame Default {
                    n310 = case shown="기본" w739 {
                      selector: w739 -> [_ w744]
                      tunnel: w742 -> [w743 w747]
                      tunnel: [w743 w746] -> w741
                      tunnel: w740 -> [_ w745]
                      frame "" {
                      }
                      frame Default {
                        n311 = Replace Array Subset(array=w747, new element=w744, index=w745) -> (w746:string[])
                      }
                    }
                  }
                }
                n312 = case shown="기본" w703 {
                  selector: w703 -> [_ w730]
                  tunnel: w710 -> [w728 w732]
                  tunnel: w708 -> [_ w729]
                  tunnel: [w728 w731] -> w714
                  frame -1 {
                  }
                  frame Default {
                    n313 = case shown="기본" w729 {
                      selector: w729 -> [_ w734]
                      tunnel: w732 -> [w733 w737]
                      tunnel: [w733 w736] -> w731
                      tunnel: w730 -> [_ w735]
                      frame "" {
                      }
                      frame Default {
                        n314 = Replace Array Subset(array=w737, new element=w734, index=w735) -> (w736:string[])
                      }
                    }
                  }
                }
                n315 = case shown="기본" w704 {
                  selector: w704 -> [_ w720]
                  tunnel: w714 -> [w718 w722]
                  tunnel: w707 -> [_ w719]
                  tunnel: [w718 w721] -> w713
                  frame -1 {
                  }
                  frame Default {
                    n316 = case shown="기본" w719 {
                      selector: w719 -> [_ w724]
                      tunnel: w722 -> [w723 w727]
                      tunnel: [w723 w726] -> w721
                      tunnel: w720 -> [_ w725]
                      frame "" {
                      }
                      frame Default {
                        n317 = Replace Array Subset(array=w727, new element=w724, index=w725) -> (w726:string[])
                      }
                    }
                  }
                }
              }
            }
            n318 = Insert Into Array(array=w649, index (row)=w644, new element=w642) -> (w646:string[][])  [unwired: 1 in]
            n319 = local write "Proc"(w646) -> ()
          }
        }
      }
      frame "종료" {
      }
      frame "에러" {
        n320 = Variant To Data(error in=w774, type=errorcluster {"status"=FALSE, "code"=0, "source"=""} ("에러 출력"), Variant=w772) -> (data=w770:errorcluster, error out=w771:errorcluster)
        n321 = call <vilib>:"Simple Error Handler.vi"("error in (no error)"=w770) -> ()  [unwired: 4 in, 5 out]
      }
    }
  }
  n322 = Merge Errors(w16, w17) -> (w15:errorcluster)
  n323 = call <vilib>:"Simple Error Handler.vi"("error in (no error)"=w15) -> ("error out"=→"error out":errorcluster)  [unwired: 4 in, 4 out]
